vi "U3 Write USB Descriptor Strings.vi"() -> (0 "error out":errorcluster)   [LabVIEW 2021]
panel:
  out "Data Array":u8[](array[numeric])
  in  "iProduct":string
  in  "iManufacturer":string
  in  "FirstFound":bool=TRUE
  in  "Address":string="1"
  out "Error Message":string
  # "Number of bytes in iManufacturer string"
  # "0x03"
  # "First character"
  # "0x00 (since Unicode)"
  # "31 characters max"
  # "31 characters max"
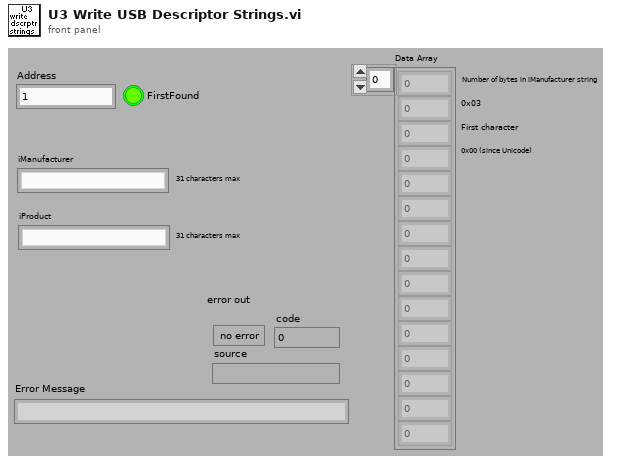
[diagram p1: front panel]
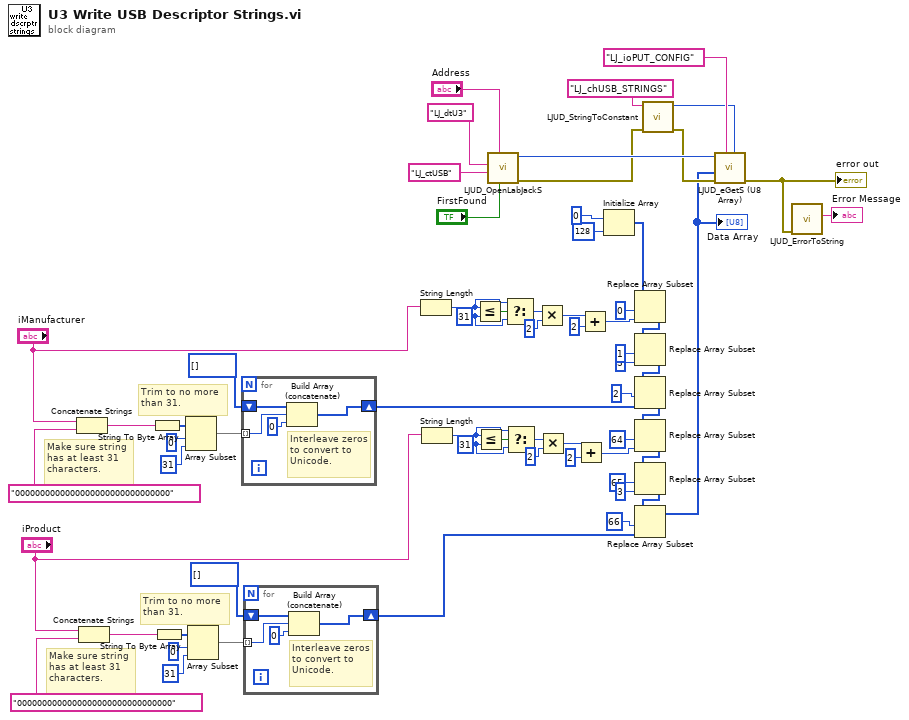
[diagram p0: block diagram]
diagram:
  w9 = 31 ("y")
  w23 = 31 ("y")
  # "Make sure string\nhas at least 31\ncharacters."
  # "Trim to no more\nthan 31."
  # "Trim to no more\nthan 31."
  # "Make sure string\nhas at least 31\ncharacters."
  n1 = Concatenate Strings("iManufacturer", "0000000000000000000000000000000") -> (w26:string)
  n2 = Concatenate Strings("iProduct", "0000000000000000000000000000000") -> (w18:string)
  n3 = String To Byte Array(string=w26) -> (unsigned byte array=w30:u8[])
  n4 = String To Byte Array(string=w18) -> (unsigned byte array=w14:u8[])
  n5 = Array Subset(array=w30, index=0 ("Array Index"), length=31 ("Array Length")) -> (w22:u8[])
  n6 = Array Subset(array=w14, index=0 ("Array Index"), length=31 ("Array Length")) -> (w19:u8[])
  n7 = for {
    tunnel: w22 -> [w67] mode=indexing
    shift-right: [w65] -> w4
    shift-left: u8[] [] -> [w64]
    # "Interleave zeros\nto convert to\nUnicode."
    n8 = Build Array (concatenate)(w64, w67, u8 0 ("Input Element")) -> (w65:u8[])
  }
  n9 = for {
    tunnel: w19 -> [w71] mode=indexing
    shift-right: [w69] -> w2
    shift-left: u8[] [] -> [w68]
    # "Interleave zeros\nto convert to\nUnicode."
    n10 = Build Array (concatenate)(w68, w71, u8 0 ("Input Element")) -> (w69:u8[])
  }
  n11 = String Length(string="iManufacturer") -> (length=w25:i32)
  n12 = String Length(string="iProduct") -> (length=w7:i32)
  n13 = Less Or Equal?(x=w25, y=w23) -> (x <= y?=w24:bool)
  n14 = Less Or Equal?(x=w7, y=w9) -> (x <= y?=w8:bool)
  n15 = call "LJUD_OpenLabJackS.vi"("FirstFound"="FirstFound", "Address"="Address", "ConnectionType"="LJ_ctUSB", "DeviceType"="LJ_dtU3") -> ("error out"=w54:errorcluster, "Handle"=w57:i32)  [unwired: 5 in, 1 out]
  n16 = Select(t=w25, s=w24, f=w23) -> (s? t:f=w13:i32)
  n17 = Select(t=w7, s=w8, f=w9) -> (s? t:f=w10:i32)
  n18 = Multiply(x=w13, y=2) -> (x*y=w3:i32)
  n19 = Multiply(x=w10, y=2) -> (x*y=w1:i32)
  n20 = Add(x=w1, y=2) -> (x+y=w34:i32)
  n21 = Add(x=w3, y=2) -> (x+y=w33:i32)
  n22 = Initialize Array(u8 0, 128 ("Dimension Size")) -> (w49:u8[])
  n23 = Replace Array Subset(array=w49, new element=w33, index=0 ("Index")) -> (w48:u8[])
  n24 = Replace Array Subset(array=w48, new element=u8 3 ("New Element/Subarray"), index=1 ("Index")) -> (w47:u8[])
  n25 = Replace Array Subset(array=w47, new element=w4, index=2 ("Index")) -> (w46:u8[])
  n26 = Replace Array Subset(array=w46, new element=w34, index=64 ("Index")) -> (w45:u8[])
  n27 = Replace Array Subset(array=w45, new element=u8 3 ("New Element/Subarray"), index=65 ("Index")) -> (w44:u8[])
  n28 = Replace Array Subset(array=w44, new element=w2, index=66 ("Index")) -> (w35:u8[])
  "Data Array" <- w35
  n29 = call "LJUD_StringToConstant.vi"("error in"=w54, "String"="LJ_chUSB_STRINGS" ("Channel")) -> ("error out"=w53:errorcluster, "Constant Number"=w52:i32)  [unwired: 8 in]
  n30 = call "LJUD_eGetS (U8 Array).vi"("Channel"=w52, "IOType"="LJ_ioPUT_CONFIG", "error in"=w53, "U8 Array Write"=w35, "Handle In"=w57) -> ("error out"=w60:errorcluster)  [unwired: 3 in, 3 out]
  "error out" <- w60
  n31 = call "LJUD_ErrorToString.vi"("error in"=w60) -> ("String"=→"Error Message":string)  [unwired: 10 in]
